vi "Instrument_Close.vi"(8 "Error In":errorcluster, 11 "PORT":string) -> (0 "Error Out":errorcluster)   [LabVIEW 2013]
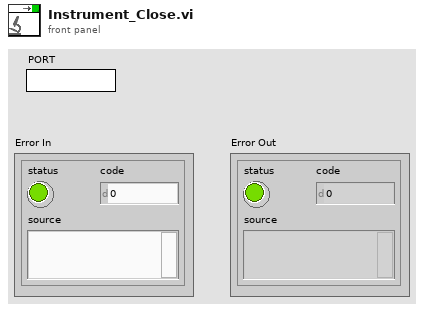
[diagram p1: front panel]
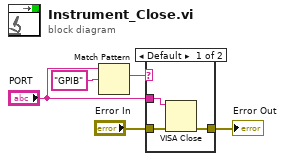
[diagram p0: block diagram]
diagram:
  n1 = Match Pattern(string="PORT", regular expression="GPIB") -> (match substring=w4:string)  [unwired: 1 in, 3 out]
  n2 = case shown="Default" w4 {
    tunnel: "Error In" -> [w8 w9]
    tunnel: [w7 w9] -> w2
    tunnel: "PORT" -> [w6 _]
    frame Default {
      n3 = VISA Close(VISA resource name=w6, error in (no error)=w8) -> (error out=w7:errorcluster)
    }
    frame "GPIB" {
    }
  }
  "Error Out" <- w2
